vi "Constructor.vi"(8 "error in (no error)":errorcluster, 11 "INL Valve Controller in":refnum<class "INL Valve Controller.lvclass">) -> (0 "error out":errorcluster, 2 "Init":bool, 3 "INL Valve Controller out":refnum<class "INL Valve Controller.lvclass">)   [LabVIEW 2011, in "INL Valve Controller.lvclass"]
uses:
  INL Valve Controller.lvclass
  INL Valve Controller.lvclass/INL Valve Controller.ctl
  <vilib>/Instr/_visa.llb/VISA Configure Serial Port (Instr).vi
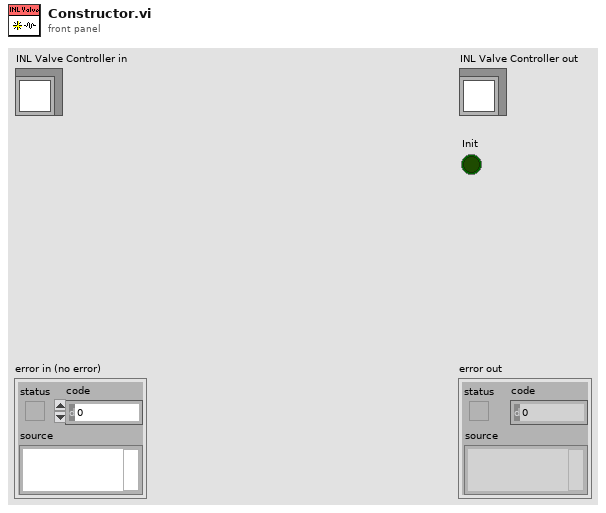
[diagram p1: front panel]
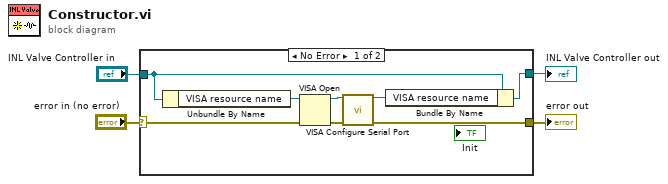
[diagram p0: block diagram]
diagram:
  n1 = case shown="No Error" "error in (no error)" {
    selector: "error in (no error)" -> [w8 w14]
    tunnel: [w7 w14] -> w3
    tunnel: [w9 w13] -> w1
    tunnel: "INL Valve Controller in" -> [w6 w13]
    frame No Error {
      n2 = Unbundle By Name(w6) -> ("VISA resource name"=w5:refnum<visa-resource-name>)
      n3 = VISA Open(error in (no error)=w8, VISA resource name=w5) -> (VISA resource name=w11:refnum<visa-resource-name>, error out=w10:errorcluster)  [unwired: 3 in]
      n4 = call-poly "VISA Configure Serial Port"("VISA resource name"=w11, "error in (no error)"=w10) -> ("VISA resource name out"=w12:refnum<visa-resource-name>, "error out"=w7:errorcluster)  [unwired: 12 in]
      n5 = Bundle By Name(cluster=w6, "VISA resource name"=w12) -> (w9:refnum<class "INL Valve Controller.lvclass">)
    }
    frame Error {
    }
  }
  "error out" <- w3
  "INL Valve Controller out" <- w1
